vi "Page Getting Started.vi"() -> ()   [LabVIEW 2018, in "Main.lvlib"]
uses:
  Main.lvlib
  Theme/Theme.lvlib
  Exit/Exit.lvlib
panel:
  in  "Listbox 3":i32(listbox)=-1 caption="Tutorials"
  in  "Listbox 2":i32(listbox)=-1 caption="Recent Projects"
  in  "New Package 2":bool
  in  "New Package":bool
  in  "New Project":bool
  # "Getting Started"
  # "Help"
  # "https://github.com/rcpacini"
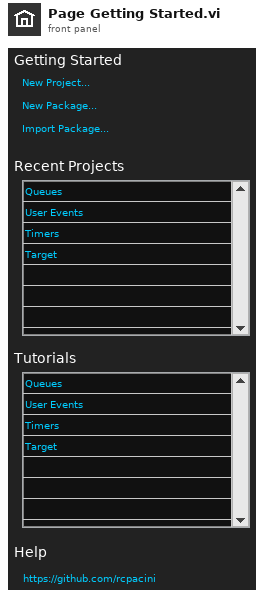
[diagram p1: front panel]
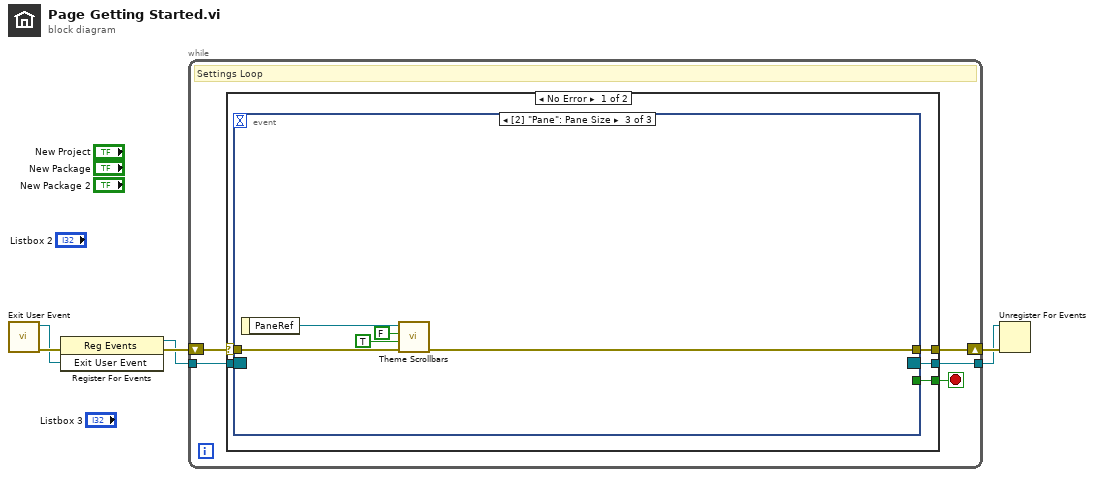
[diagram p0: block diagram]
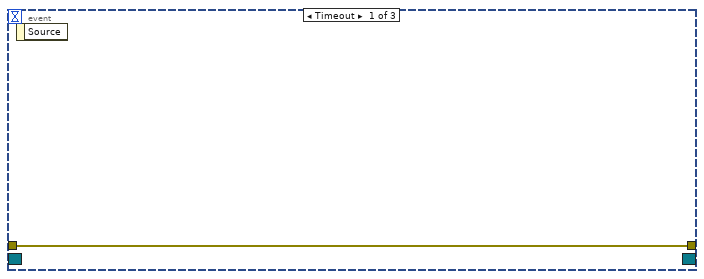
[diagram p2: hidden frame]
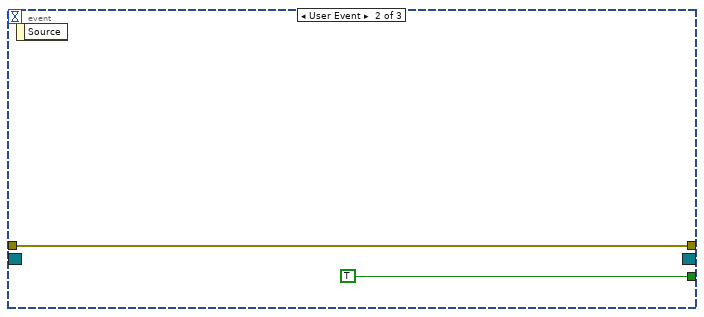
[diagram p3: hidden frame]
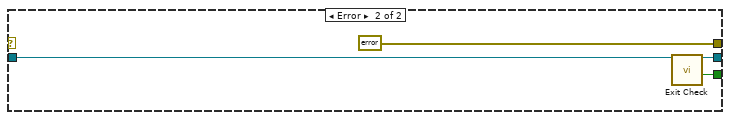
[diagram p4: hidden frame]
diagram:
  n1 = call "Exit User Event.vi"() -> ("error out"=w5:errorcluster, "Exit User Event"=w4:refnum<user-event>)  [unwired: 10 in]
  n2 = register-events(error in=w5, w4) -> (reference out=w3:refnum<event-registration>, error out=w6:errorcluster)  [unwired: 1 in]
  n3 = while {
    tunnel: w3 -> [w10]
    shift-right: [w9] -> w2
    shift-left: w6 -> [w11]
    tunnel: [w7] -> w1
    stop <- w8 stop-if-true
    # "Settings Loop"
    n4 = case shown="No Error" w11 {
      selector: w11 -> [w16 _]
      tunnel: w10 -> [w15 w25]
      tunnel: [w14 errorcluster {"status"=FALSE, "code"=0, "source"=""} ("error IO")] -> w9
      tunnel: [w12 w26] -> w8
      tunnel: [w13 w25] -> w7
      frame No Error {
        n5 = event shown="[2] \"Pane\": Pane Size" {
          selector: w15 -> [_ _ _]
          dyn-events: [_ _ _] -> w13
          timeout: _ -> [_ _ _]
          tunnel: w16 -> [w17 w19 w24]
          tunnel: [w17 w19 w23] -> w14
          tunnel: [_ TRUE _] -> w12
          event Timeout {
            n6 = event-data() -> ()  [unwired: 1 in, 1 out]
          }
          event User Event {
            n7 = event-data() -> ()  [unwired: 1 in, 1 out]
          }
          event Pane Size {
            n8 = event-data() -> ("PaneRef"=w22:refnum<vi>)  [unwired: 1 in]
            n9 = call "Theme Scrollbars.vi"("error in (no error)"=w24, "Vertical Scrollbar? (T)"=TRUE, "Horizontal Scrollbar? (T)"=FALSE, "Pane in"=w22) -> ("error out"=w23:errorcluster)  [unwired: 6 in, 1 out]
          }
        }
      }
      frame Error {
        n10 = call "Exit Check.vi"() -> ("Exit?"=w26:bool)  [unwired: 10 in, 1 out]
      }
    }
  }
  n11 = Unregister For Events(event registration refnum=w1, error in=w2) -> ()  [unwired: 1 out]
